vi "New motor Control no PID.vi"(0 "Encoder 0":dbl, 1 "Encoder 1":dbl, 2 "Encoder 2":dbl, 3 "xTargetSpeed":dbl, 4 "yTargetSpeed":dbl, 5 "wTargetSpeed":dbl) -> (14 "M2":dbl format="%.2f", 15 "M0":dbl format="%.2f", 16 "M1":dbl format="%.2f")   [LabVIEW 2018]
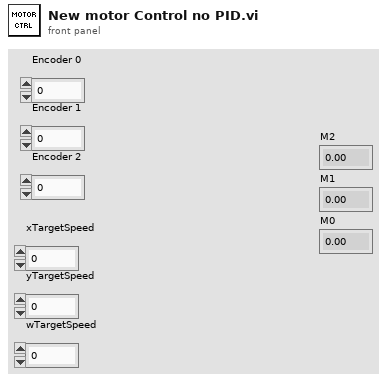
[diagram p1: front panel]
types:
  T1 = cluster{"Encoder 0":dbl, "Encoder 1":dbl, "Encoder 2":dbl}
  T2 = cluster{"proportional gain (Kc)":dbl, "integral time (Ti, min)":dbl, "derivative time (Td, min)":dbl}
  T3 = cluster{"xSpeed":dbl, "ySpeed":dbl, "wSpeed":dbl}
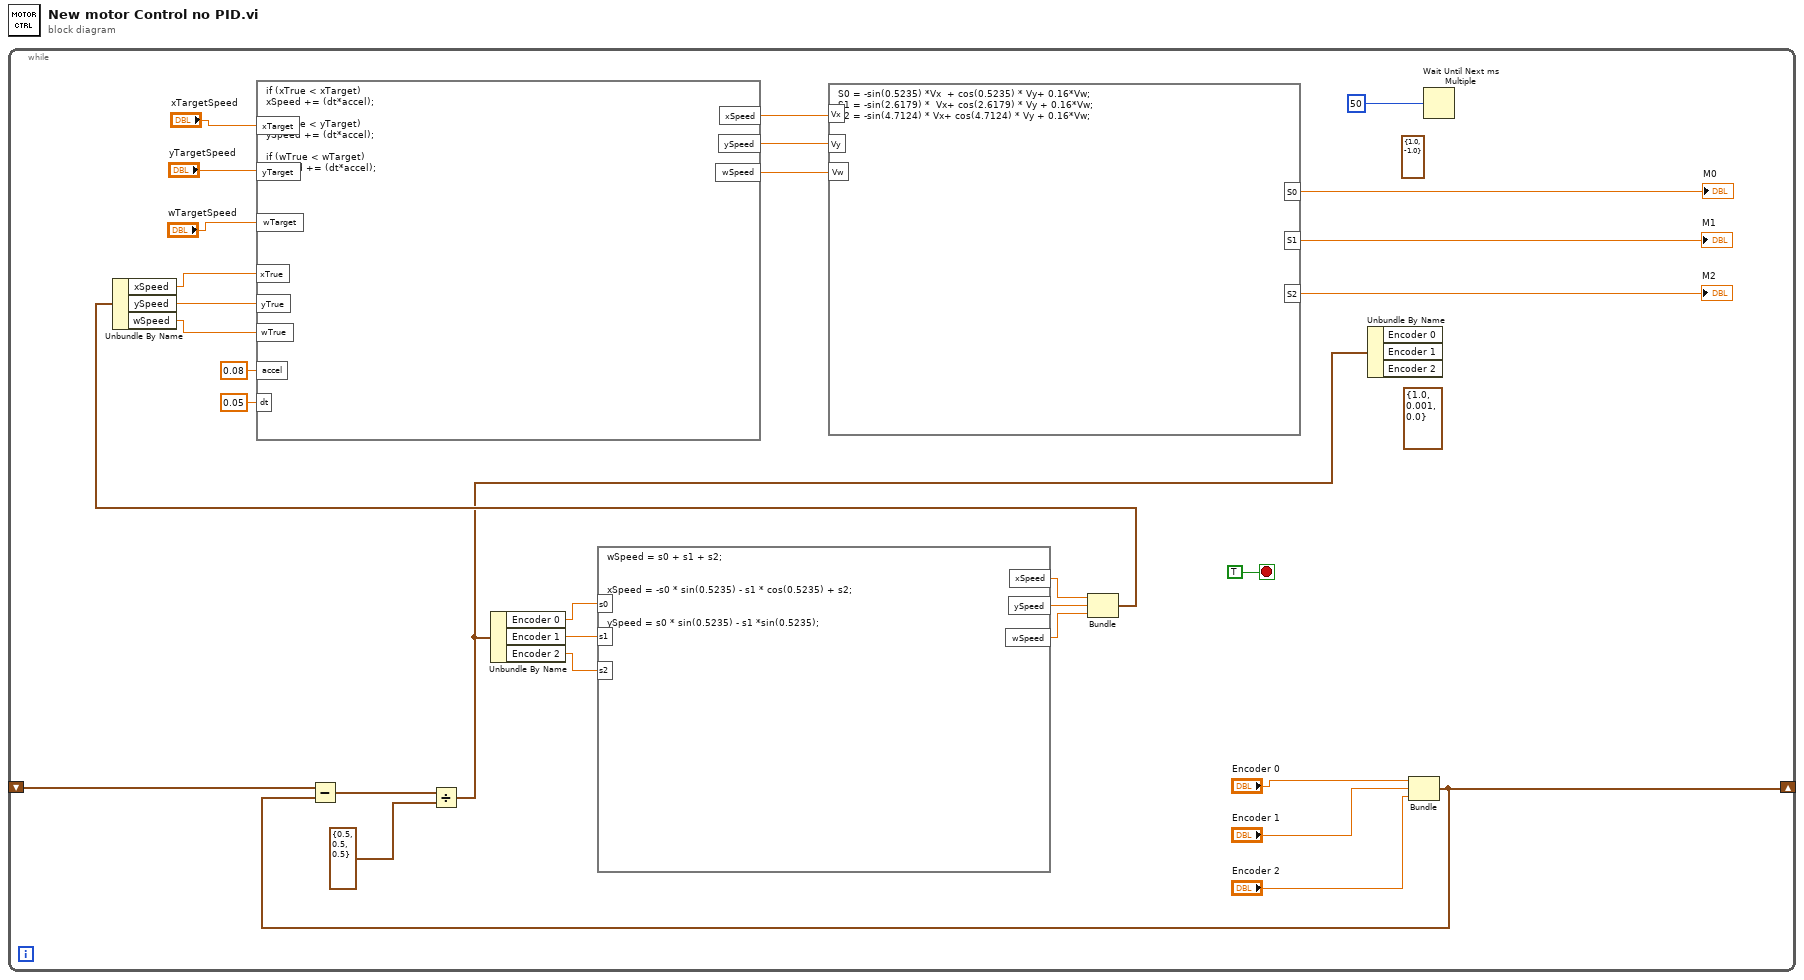
[diagram p0: block diagram]
diagram:
  n1 = while {
    shift-right: [w26] -> _
    shift-left: _ -> [w27]
    stop <- TRUE stop-if-true
    (unwired) cluster{"output high":dbl, "output low":dbl} {"output high"=1.0, "output low"=-1.0} ("output range")
    (unwired) T2 {"proportional gain (Kc)"=1.0, "integral time (Ti, min)"=0.001, "derivative time (Td, min)"=0.0} ("PID gains")
    n2 = Bundle("Encoder 0"="Encoder 0", "Encoder 1"="Encoder 1", "Encoder 2"="Encoder 2") -> (w26:T1)  [unwired: 1 in]
    n3 = Subtract(x=w27, y=w26) -> (x-y=w25:T1)
    n4 = Divide(x=w25, y=T1 {"Encoder 0"=0.5, "Encoder 1"=0.5, "Encoder 2"=0.5}) -> (x/y=w7:T1)
    n5 = Unbundle By Name(w7) -> ("Encoder 0"=w22:dbl, "Encoder 1"=w23:dbl, "Encoder 2"=w21:dbl)
    n6 = formula code="wSpeed = s0 + s1 + s2;\n\n\nxSpeed = -s0 * sin(0.5235) - s1 * cos(0.5235) + s2;\n\n\nySpeed = s0 * sin(0.5235) - s1 *sin(0.5235);"("s0"=w22, "s1"=w23, "s2"=w21) -> ("xSpeed"=w19:dbl, "ySpeed"=w20:dbl, "wSpeed"=w18:dbl)
    n7 = Bundle("xSpeed"=w19, "ySpeed"=w20, "wSpeed"=w18) -> (w17:T3)  [unwired: 1 in]
    n8 = Unbundle By Name(w17) -> ("xSpeed"=w16:dbl, "ySpeed"=w15:dbl, "wSpeed"=w14:dbl)
    n9 = formula code="if (xTrue < xTarget)\nxSpeed += (dt*accel);\n\nif (yTrue < yTarget)\nySpeed += (dt*accel);\n\nif (wTrue < wTarget)\nwSpeed += (dt*accel);"("xTarget"="xTargetSpeed", "yTarget"="yTargetSpeed", "wTarget"="wTargetSpeed", "xTrue"=w16, "yTrue"=w15, "wTrue"=w14, "accel"=0.08 ("input variable"), "dt"=0.05 ("input variable")) -> ("xSpeed"=w10:dbl, "ySpeed"=w9:dbl, "wSpeed"=w8:dbl)
    n10 = formula code="S0 = -sin(0.5235) *Vx  + cos(0.5235) * Vy+ 0.16*Vw;\nS1 = -sin(2.6179) *  Vx+ cos(2.6179) * Vy + 0.16*Vw;\nS2 = -sin(4.7124) * Vx+ cos(4.7124) * Vy + 0.16*Vw;"("Vx"=w10, "Vy"=w9, "Vw"=w8) -> ("S0"=→"M0":dbl, "S1"=→"M1":dbl, "S2"=→"M2":dbl)
    n11 = Unbundle By Name(w7) -> ()  [unwired: 3 out]
    n12 = Wait Until Next ms Multiple(millisecond multiple=u32 50) -> ()  [unwired: 1 out]
  }
